vi "clear Session Data.vi"(0 "FPGA Serial In":refnum<class "FPGA Serial Session.lvclass">, 11 "error in":errorcluster) -> (4 "FPGA Serial Out":refnum<class "FPGA Serial Session.lvclass">, 15 "error out":errorcluster)   [LabVIEW 2015, in "FPGA Serial Session.lvclass"]
doc: "OVERRIDE VI\nPlaceholder for decendant classes to clear session information and close references."
uses:
  FPGA Serial Session.lvclass
  Raw FPGA/FPGA Session.lvclass
  FPGA Serial Session.lvclass/FPGA Serial Session.ctl
  Reusable/Session APIs/Text Communication/Text Device Session.lvclass
  <userlib>/_Session Fwk/Session - Root.lvclass
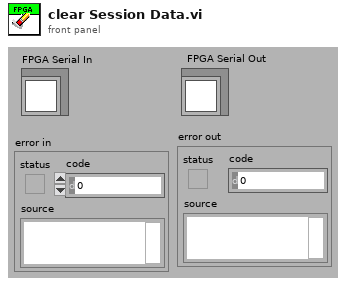
[diagram p1: front panel]
types:
  T1 = typedef "Session - Root.lvclass/Session Handle.ctl" = refnum<data-value>
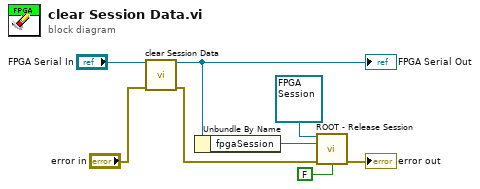
[diagram p0: block diagram]
diagram:
  n1 = call-parent "clear Session Data.vi"("OBJ - Measurement Session in"="FPGA Serial In", "error in"="error in") -> ("OBJ - Measurement Session out"=w3:refnum<class "FPGA Serial Session.lvclass">, "error out"=w1:errorcluster)  [unwired: 12 in]
  "FPGA Serial Out" <- w3
  n2 = Unbundle By Name(w3) -> ("fpgaSession"=w8:T1)
  n3 = call <userlib>:"ROOT - Release Session.vi"("OBJ - Session in"=refnum<class "FPGA Session.lvclass"> refnum ("FPGA Session"), "Session Handle in"=w8, "error in (no error)"=w1, "force destroy? (F)"=FALSE) -> ("error out"=→"error out":errorcluster)  [unwired: 10 in, 1 out]
